vi "ValidateTargetParameter.vi"(8 "error in":errorcluster, 9 "Supported Devices":u32[](array[numeric]), 10 "TargetInfoHistory":T1 {"IPTargetList"."Target RT Info List"."ProdID" format="%.0x"; "USBTargetList"."Target RT Info List"."ProdID" format="%.0x"; "WiFiTargetList"."Target RT Info List"."ProdID" format="%.0x"; "GenericTargetList"."Target RT Info List"."ProdID" format="%.0x"}, 11 "UI Ref Cluster":T4) -> (0 "error out":errorcluster, 2 "Error Message":string, 3 "UI Ref Cluster Out":T4)   [LabVIEW 2021, in "myRIOMetaDataObj.lvclass"]
uses:
  myRIOMetaDataObj.lvclass
  WizardUIRef.ctl
  AvailableTargets.ctl
  TargetInfoHistory.ctl
  TargetListInfo.ctl
  <resource>/myRIO/Target Info.ctl
  <vilib>/Utility/error.llb/DialogType.ctl
  InternalErrorCodes.vi
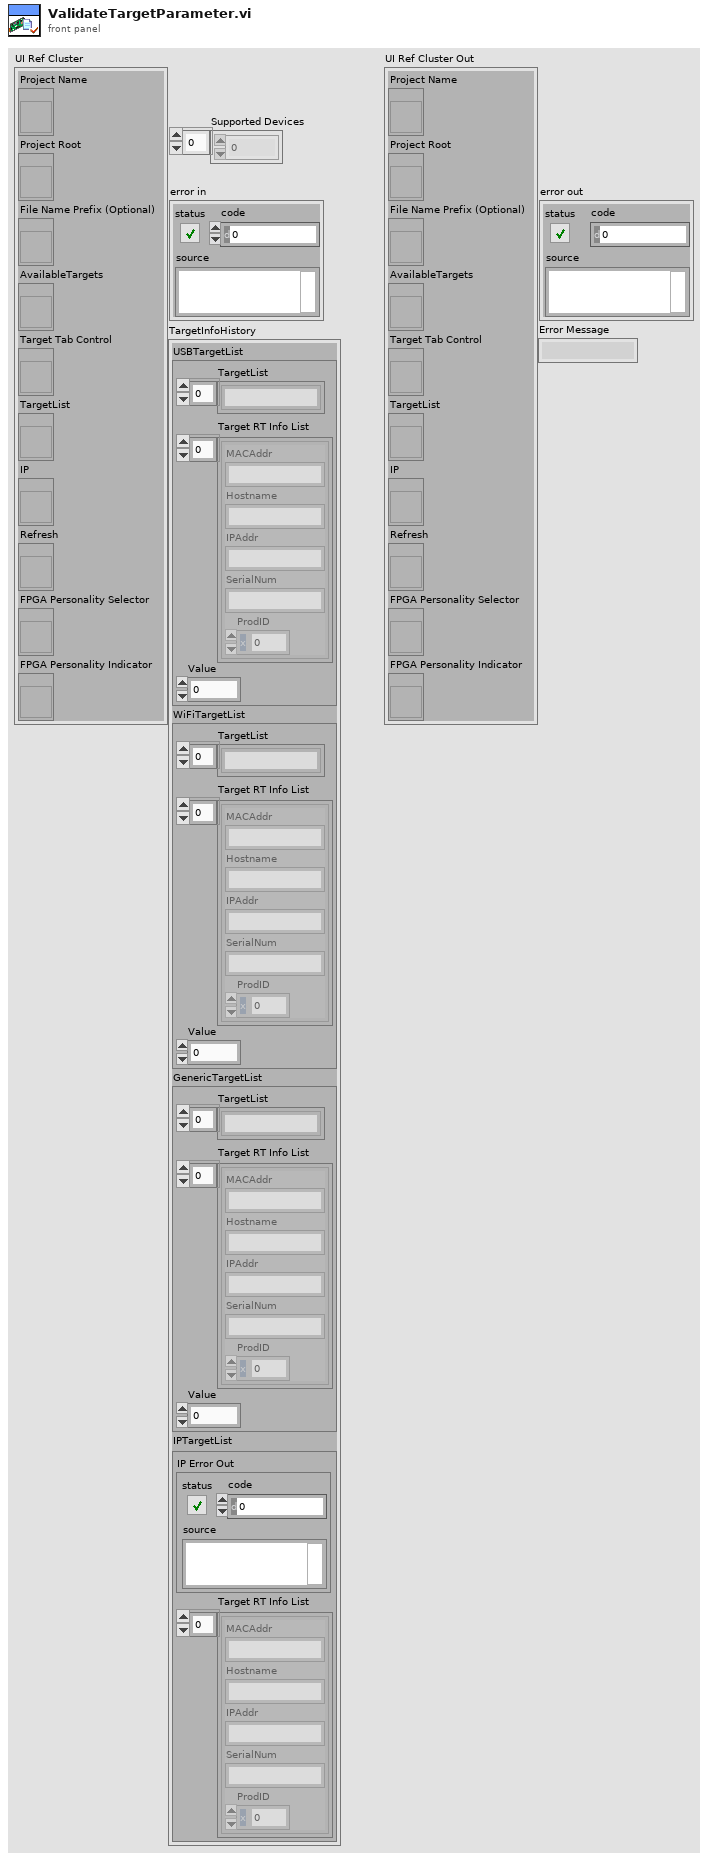
[diagram p1: front panel]
types:
  T1 = typedef "myRIOMetaDataObj.lvclass/TargetInfoHistory.ctl" = cluster{"USBTargetList":T2, "WiFiTargetList":T2, "GenericTargetList":T2, "IPTargetList":cluster{"IP Error Out":errorcluster, "Target RT Info List":T3[]}}
  T2 = typedef "myRIOMetaDataObj.lvclass/TargetListInfo.ctl" = cluster{"TargetList":string[], "Value":i32, "Target RT Info List":T3[]}
  T3 = typedef "Target Info.ctl" = cluster{"MACAddr":string, "Hostname":string, "IPAddr":string, "SerialNum":string, "ProdID":u32}
  T4 = typedef "myRIOMetaDataObj.lvclass/WizardUIRef.ctl" = cluster{"Project Name":refnum<vi>, "Project Root":refnum<vi>, "File Name Prefix (Optional)":refnum<vi>, "AvailableTargets":refnum<vi>, "Target Tab Control":refnum<vi>, "TargetList":refnum<vi>, "IP":refnum<vi>, "Refresh":refnum<vi>, "FPGA Personality Selector":refnum<vi>, "FPGA Personality Indicator":refnum<vi>}
  T5 = typedef "myRIOMetaDataObj.lvclass/AvailableTargets.ctl" = enum32{"USBTarget", "WifiTarget", "NoSpecificTarget", "TargetIP"}
  T6 = typedef "DialogType.ctl" = u16
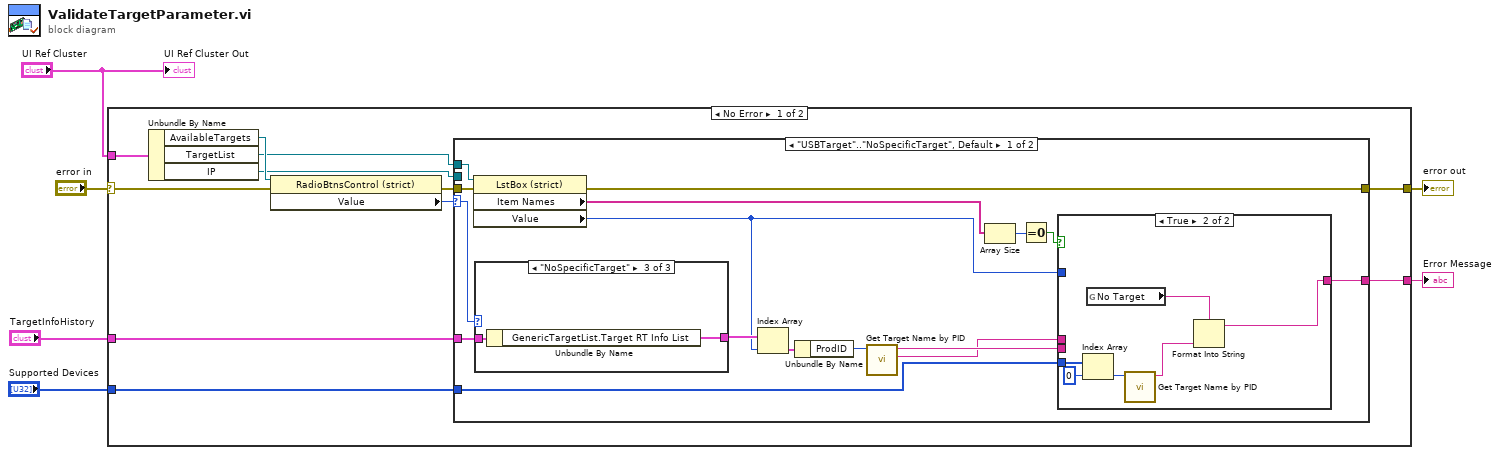
[diagram p0: block diagram]
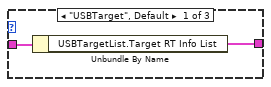
[diagram p2: hidden frame]
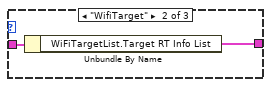
[diagram p3: hidden frame]
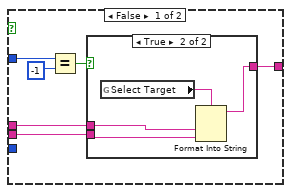
[diagram p4: hidden frame]
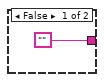
[diagram p5: hidden frame]
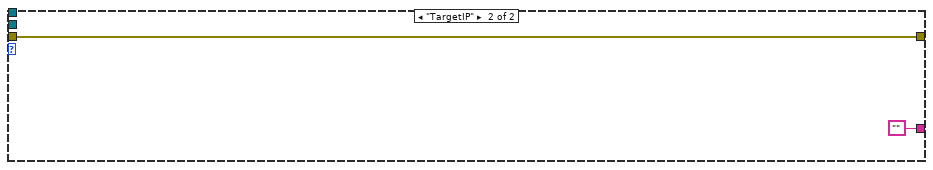
[diagram p6: hidden frame]
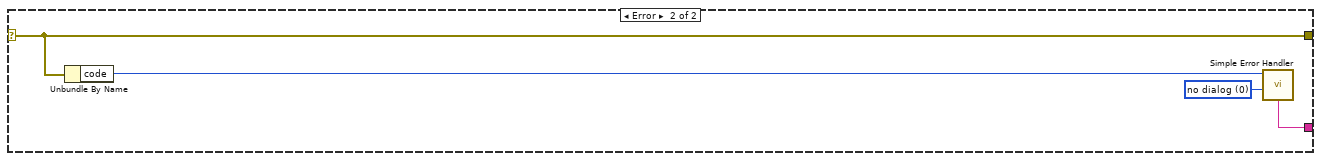
[diagram p7: hidden frame]
diagram:
  n1 = case shown="No Error" "error in" {
    selector: "error in" -> [w15 w59]
    tunnel: [w10 w59] -> w5
    tunnel: [w11 w60] -> w3
    tunnel: "UI Ref Cluster" -> [w17 _]
    tunnel: "TargetInfoHistory" -> [w8 _]
    tunnel: "Supported Devices" -> [w7 _]
    frame No Error {
      n2 = Unbundle By Name(w17) -> ("AvailableTargets"=w16:refnum<vi>, "TargetList"=w13:refnum<vi>, "IP"=w12:refnum<vi>)
      n3 = property class="RadioBtnsControl (strict)"(reference=w16, error in=w15) -> (error out=w14:errorcluster, "Value"=w9:T5)  [unwired: 1 out]
      n4 = case shown="\"USBTarget\"..\"NoSpecificTarget\", Default" w9 {
        selector: w9 -> [w26 _]
        tunnel: w14 -> [w32 w58]
        tunnel: w13 -> [w33 _]
        tunnel: w12 -> [_ _]
        tunnel: [w28 ""] -> w11
        tunnel: [w27 w58] -> w10
        tunnel: w8 -> [w25 _]
        tunnel: w7 -> [w19 _]
        frame "USBTarget".."NoSpecificTarget", Default {
          n5 = property class="LstBox (strict)"(reference=w33, error in=w32) -> (error out=w27:errorcluster, "Item Names"=w31:string[], "Value"=w22:i32)  [unwired: 1 out]
          n6 = case shown="\"NoSpecificTarget\"" w26 {
            tunnel: w25 -> [w35 w37 w39]
            tunnel: [w34 w36 w38] -> w23
            frame "USBTarget", Default {
              n7 = Unbundle By Name(w35) -> ("USBTargetList.Target RT Info List"=w34:T3[])
            }
            frame "WifiTarget" {
              n8 = Unbundle By Name(w37) -> ("WiFiTargetList.Target RT Info List"=w36:T3[])
            }
            frame "NoSpecificTarget" {
              n9 = Unbundle By Name(w39) -> ("GenericTargetList.Target RT Info List"=w38:T3[])
            }
          }
          n10 = Index Array(array=w23, index=w22) -> (element=w24:T3)
          n11 = Unbundle By Name(w24) -> ("ProdID"=w21:u32)
          n12 = call <vilib>:"Get Target Name by PID.vi"("Device Model"=w21) -> ("Article"=w18:string, "Device Model Str"=w20:string)  [unwired: 9 in]
          n13 = Array Size(array=w31) -> (size(s)=w30:i32)
          n14 = Equal To 0?(x=w30) -> (x = 0?=w29:bool)
          n15 = case shown="True" w29 {
            tunnel: [w42 w55] -> w28
            tunnel: w22 -> [w45 _]
            tunnel: w20 -> [w41 _]
            tunnel: w19 -> [_ w54]
            tunnel: w18 -> [w40 _]
            frame False {
              n16 = Equal?(x=w45, y=-1) -> (x = y?=w43:bool)
              n17 = case shown="True" w43 {
                tunnel: ["" w49] -> w42
                tunnel: w41 -> [_ w48]
                tunnel: w40 -> [_ w47]
                frame False {
                }
                frame True {
                  n18 = global read "InternalErrorCodes.vi" "Select Target"() -> (w50:string)
                  n19 = Format Into String(format string=w50, w47, w48) -> (resulting string=w49:string)  [unwired: 2 in, 1 out]
                }
              }
            }
            frame True {
              n20 = Index Array(array=w54, index=0) -> (element=w52:u32)
              n21 = global read "InternalErrorCodes.vi" "No Target"() -> (w56:string)
              n22 = call <vilib>:"Get Target Name by PID.vi"("Device Model"=w52) -> ("Device Model Str"=w51:string)  [unwired: 9 in, 1 out]
              n23 = Format Into String(format string=w56, w51) -> (resulting string=w55:string)  [unwired: 2 in, 1 out]
            }
          }
        }
        frame "TargetIP" {
        }
      }
    }
    frame Error {
      w61 = T6 0 items=["no dialog", "OK message", "continue or stop message", "OK message + warnings", "continue/stop + warnings"] ("type of dialog (OK msg:1)")
      n24 = Unbundle By Name(w59) -> ("code"=w62:i32)
      n25 = call <vilib>:"Simple Error Handler.vi"("error code (no error:0)"=w62, "type of dialog (OK msg:1)"=w61) -> ("message"=w60:string)  [unwired: 3 in, 4 out]
    }
  }
  "error out" <- w5
  "Error Message" <- w3
  "UI Ref Cluster Out" <- "UI Ref Cluster"
